vi "FPGA_RTDS_PCC_v02b_clean.vi"() -> ()   [LabVIEW 2015]
uses:
  Analog Measurements Cluster.ctl
  Reactive Power Cluster.ctl
  Real Power Cluster.ctl
  <vilib>/Platform/TimedLoop/XDataNode/timing_clust.ctl
  <vilib>/Platform/TimedLoop/XDataNode/nitl_modes.ctl
  <vilib>/Platform/TimedLoop/XDataNode/wakeup.ctl
  <vilib>/rvi/FXPMathLib/basic elements/FxpIntAccumulator/subVIs/nifxpmath_IntAccumulator_SimConfig.ctl
  <vilib>/rvi/FXPMathLib/FxpSinAndCos/subVIs/nifxpmath_SinAndCos_SimConfig.ctl
  <vilib>/rvi/FXPMathLib/FxpSqrt/subVIs/nifxpmath_Sqrt_SimConfig.ctl
  <vilib>/fxp/LVFixedPointOverflowPolicyTypeDef.ctl
  <vilib>/rvi/Emulation/niFpgaGetClockAttributes.vi
  <vilib>/rvi/Emulation/niFpgaSctlEmulationGetInTimedLoop.vi
  <vilib>/rvi/Emulation/niFpgaEmulationReportErrorSimple.vi
  <vilib>/rvi/eio/common/nirviEmuTemplateMethod_errors.vi
  <vilib>/rvi/Emulation/niFpgaProcessEmulError.vi
  <vilib>/rvi/Emulation/niFpgaCriticalErrorInLSC.vi
  <vilib>/rvi/Analysis/common/codeGenErrors/XNode/niFpgaXNodeCodeGenErrorHandle.vi
  <vilib>/rvi/FXPMathLib/basic elements/FxpIntAccumulator/simVIs/DllFxpIntAccumulator_sub.vi
  <vilib>/rvi/FXPMathLib/FxpSqrt/simVIs/DllSqrtTemp_sub.vi
  <vilib>/rvi/FXPMathLib/FxpSinAndCos/simVIs/DllFxpSinAndCosTemp_sub.vi
  <vilib>/eio/EIONode/EIONode.xnode
  <vilib>/rvi/Analysis/measure/dc-rms/XNode/niFpgaDC-RMS.xnode
  <vilib>/Platform/TimedLoop/XDataNode/XDataNode.xnode
  <vilib>/rvi/FXPMathLib/basic elements/FxpIntAccumulator/XNode/nifxpmath_IntAccumulator.xnode
  <vilib>/rvi/FXPMathLib/FxpMul/XNode/nifxpmath_Multiplier.xnode
  <vilib>/rvi/FXPMathLib/FxpSqrt/XNode/nifxpmath_Sqrt.xnode
  <vilib>/rvi/FXPMathLib/FxpSinAndCos/XNode/nifxpmath_SinAndCos.xnode
  <vilib>/rvi/Analysis/measure/mean-var-std/XNode/niFpgaMean-Var-Std.xnode
  <vilib>/Platform/TimedLoop/XDataNode/XDNodeRunTimeDep.lvlib
  <vilib>/rvi/FXPMathLib/sim/FxpSim.dll
panel:
  in  "close threshold":fxp<+,27,5>=0.09999990463256836 format="%#_24g"
  out "RMS Voltage in Range (resync)":bool
  out "RMS Time":u32
  in  "RMS Loop Time":u32=1500 caption="Count(Ticks)"
  out "Grid I RMS":fxp<+,27,5>
  out "output rms valid":bool
  in  "RMS reset":bool
  in  "Vgrid RMS constant (off grid)":fxp<+,27,5>=0.1399998664855957
  out "Microgrid RMS":fxp<+,27,5>
  out "Grid RMS":fxp<+,27,5>
  out "Mean Computation Valid":bool
  in  "Mean Reset":bool
  out "Phase Diff":fxp<+/-,33,2>
  out "cos(x)":fxp<+/-,16,2>
  out "sin(x)":fxp<+/-,16,2>
  out "Real Power (from mean)":T1
  in  "Computation Loop Time (uSec)":u32=10 caption="Count(uSec)"
  out "Mean Computation Timing Error":bool
  out "Real Power (from angle)":T1
  out "Reactive Power":T2
  in  "Data Acquisition Loop Time (uSec)":u32=10 caption="Count(uSec)"
  out "Data Acquisition Timing Error":bool
  out "Va grid":fxp<+/-,16,5>
  out "Vb grid":fxp<+/-,16,5>
  out "Vc grid":fxp<+/-,16,5>
  out "Ia":fxp<+/-,16,5>
  out "Ib":fxp<+/-,16,5>
  out "Ic":fxp<+/-,16,5>
  out "Phase angle error":fxp<+,32,1>
  out "Freq error":fxp<+,32,8>
  in  "Resync Loop Time":u32=1500 caption="Count(Ticks)"
  out "Resync Time":u32
  in  "Freq constant":fxp<+,32,8>
  out "Switch Closed?":bool
  out "Voltage error\n(on grid)":fxp<+,31,9>
  in  "Enable Resync":bool
  out "Close Switch":bool
  in  "Phase angle constant":fxp<+,32,1>=0.049999999813735485
  out "Open Switch":bool
  in  "MG_SW_constant":fxp<+/-,24,5>=4.0
  in  "Voltage constant (on grid)":fxp<+/-,28,7>=0.26999998092651367
  in  "Vgrid RMS constant (on grid)":fxp<+,27,9>=2.770000457763672
  in  "Enable Switching":bool
  out "Microgrid switch signal":fxp<+/-,24,5>
  in  "Manually Close":bool
  in  "Manually Open":bool
  out "Current\npll phase":fxp<+/-,32,1> format="%.32g"
  out "Current \nfrequency":fxp<+,32,8> format="%.27g"
  in  "PLL Loop Time":u32=1500 caption="Count(Ticks)"
  out "PLL Time MG":u32
  in  "Ki":fxp<+,16,9>=1.0
  in  "Kp":fxp<+,16,6>=0.0146484375
  in  "Ka":fxp<+,16,9>=1.0 format="%#_10g"
  out "Microgrid\npll phase":fxp<+/-,32,1> format="%.32g"
  out "Microgrid \nfrequency":fxp<+,32,8> format="%.27g"
  out "Grid\npll phase":fxp<+/-,32,1> format="%.32g"
  out "Grid \nFrequency":fxp<+,32,8> format="%.27g"
  in  "PLL dt":fxp<+,24,-5>=9.999983012676239e-05 format="%#_28g"
  in  "Reset PLL":bool
  in  "LPF Alpha":sgl[](array[numeric])=[0.19, 0.19, 0.19, 0.1, 0.1, 0.1, 0.1, 0.1, 0.1]
  in  "LPF enable":bool=TRUE
  out "Grid Iabc":T3
  out "Grid Vabc":T4
  out "Microgrid Vabc":T4
  in  "Count(Ticks)":u32=1500
  out "Loop rate":u32
  out "RMS Computation Valid":bool
  out "RMS Computation Timing Error":bool
  out "Analog rms output":T5
  # "Logic RMS Computation"
  # "Power Computation"
  # "Data Acquisition"
  # "RMS Computation"
  # "PLL Calculations"
  # "Low Pass Filter"
  # "RMS Computation"
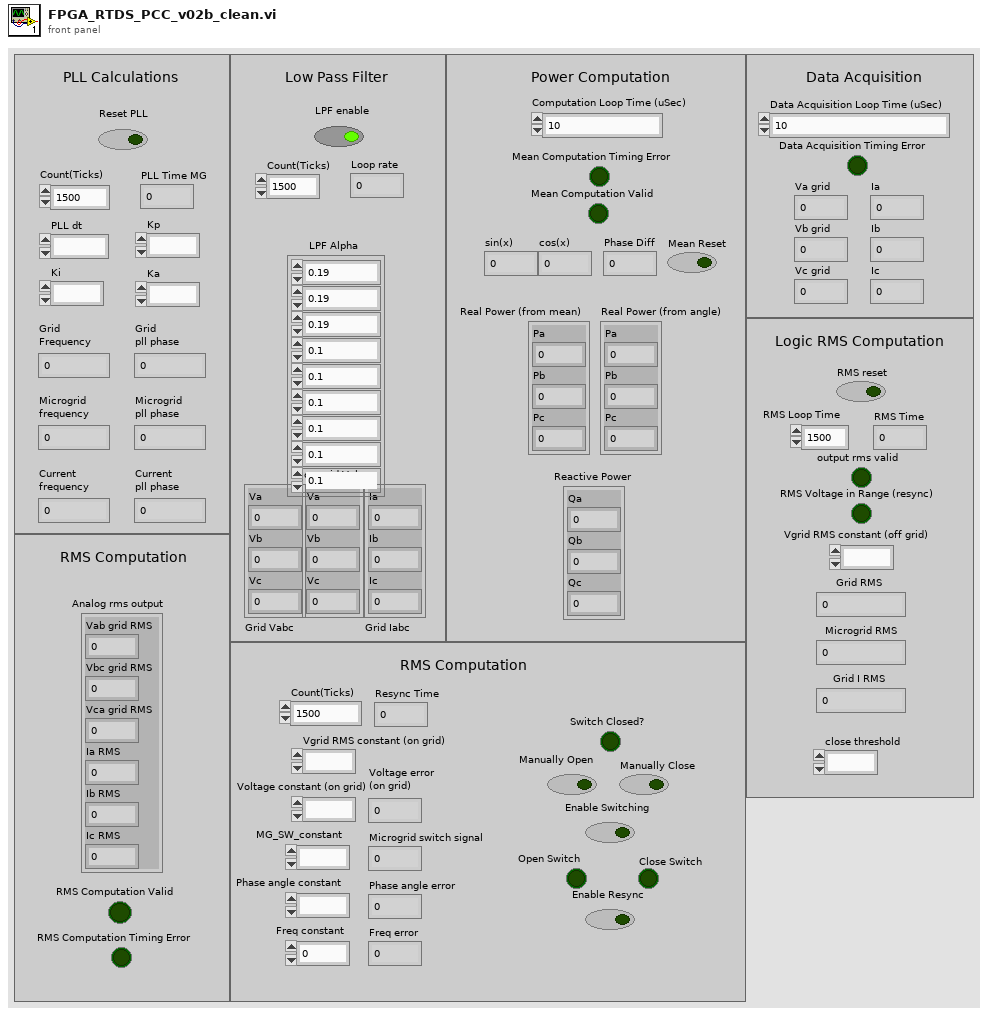
[diagram p1: front panel]
types:
  T1 = typedef "Real Power Cluster.ctl" = cluster{"Pa":fxp<+/-,32,10>, "Pb":fxp<+/-,32,10>, "Pc":fxp<+/-,32,10>}
  T2 = typedef "Reactive Power Cluster.ctl" = cluster{"Qa":fxp<+/-,46,10>, "Qb":fxp<+/-,46,10>, "Qc":fxp<+/-,46,10>}
  T3 = cluster{"Ia":fxp<+/-,24,5>, "Ib":fxp<+/-,24,5>, "Ic":fxp<+/-,24,5>}
  T4 = cluster{"Va":fxp<+/-,18,4>, "Vb":fxp<+/-,18,4>, "Vc":fxp<+/-,18,4>}
  T5 = typedef "Analog Measurements Cluster.ctl" = cluster{"Vab grid RMS":fxp<+,16,5>, "Vbc grid RMS":fxp<+,16,5>, "Vca grid RMS":fxp<+,16,5>, "Ia RMS":fxp<+,16,5>, "Ib RMS":fxp<+,16,5>, "Ic RMS":fxp<+,16,5>}
  T6 = typedef "XDNodeRunTimeDep.lvlib/timing_clust.ctl" = cluster{"Expected End [f-1]":u64, "Actual End [f-1]":u64, "Finished Late? [f-1]":bool, "Expected End [i-1]":u64, "Actual End [i-1]":u64, "Finished Late? [i-1]":bool, "Expected Start [i]":u64, "Actual Start [i]":u64, "Expected Start [f]":u64, "Actual Start [f]":u64, "Source Name":string, "Structure Name":string, "Period":i64, "Deadline":i64, "Offset":i64, "Start":i64, "Priority":i32, "Timeout":i32, "Mode":T7, "Wakeup Reason":T8, "Error":errorcluster, "Source Type":string, "Secondary Source Type":string, "Global End Time":u64, "Global Start Time":u64, "Frame Duration":u64, "Iteration Duration":u64, "Assigned CPU":i32, "I/O Scan Engine Mode":u32}
  T7 = typedef "XDNodeRunTimeDep.lvlib/nitl_modes.ctl" = enum32{"No Change", "Process missed periods, maintain original phase", "Discard missed periods, maintain original phase", "Process missed periods, ignore original phase", "Discard missed periods, ignore original phase"}
  T8 = typedef "XDNodeRunTimeDep.lvlib/wakeup.ctl" = enum32{"Normal", "Aborted", "Asynchronous wakeup", "Timing source error", "Timed loop error", "Timeout"}
  T9 = cluster{"filtered x":sgl, "filtered x":sgl, "filtered x":sgl}
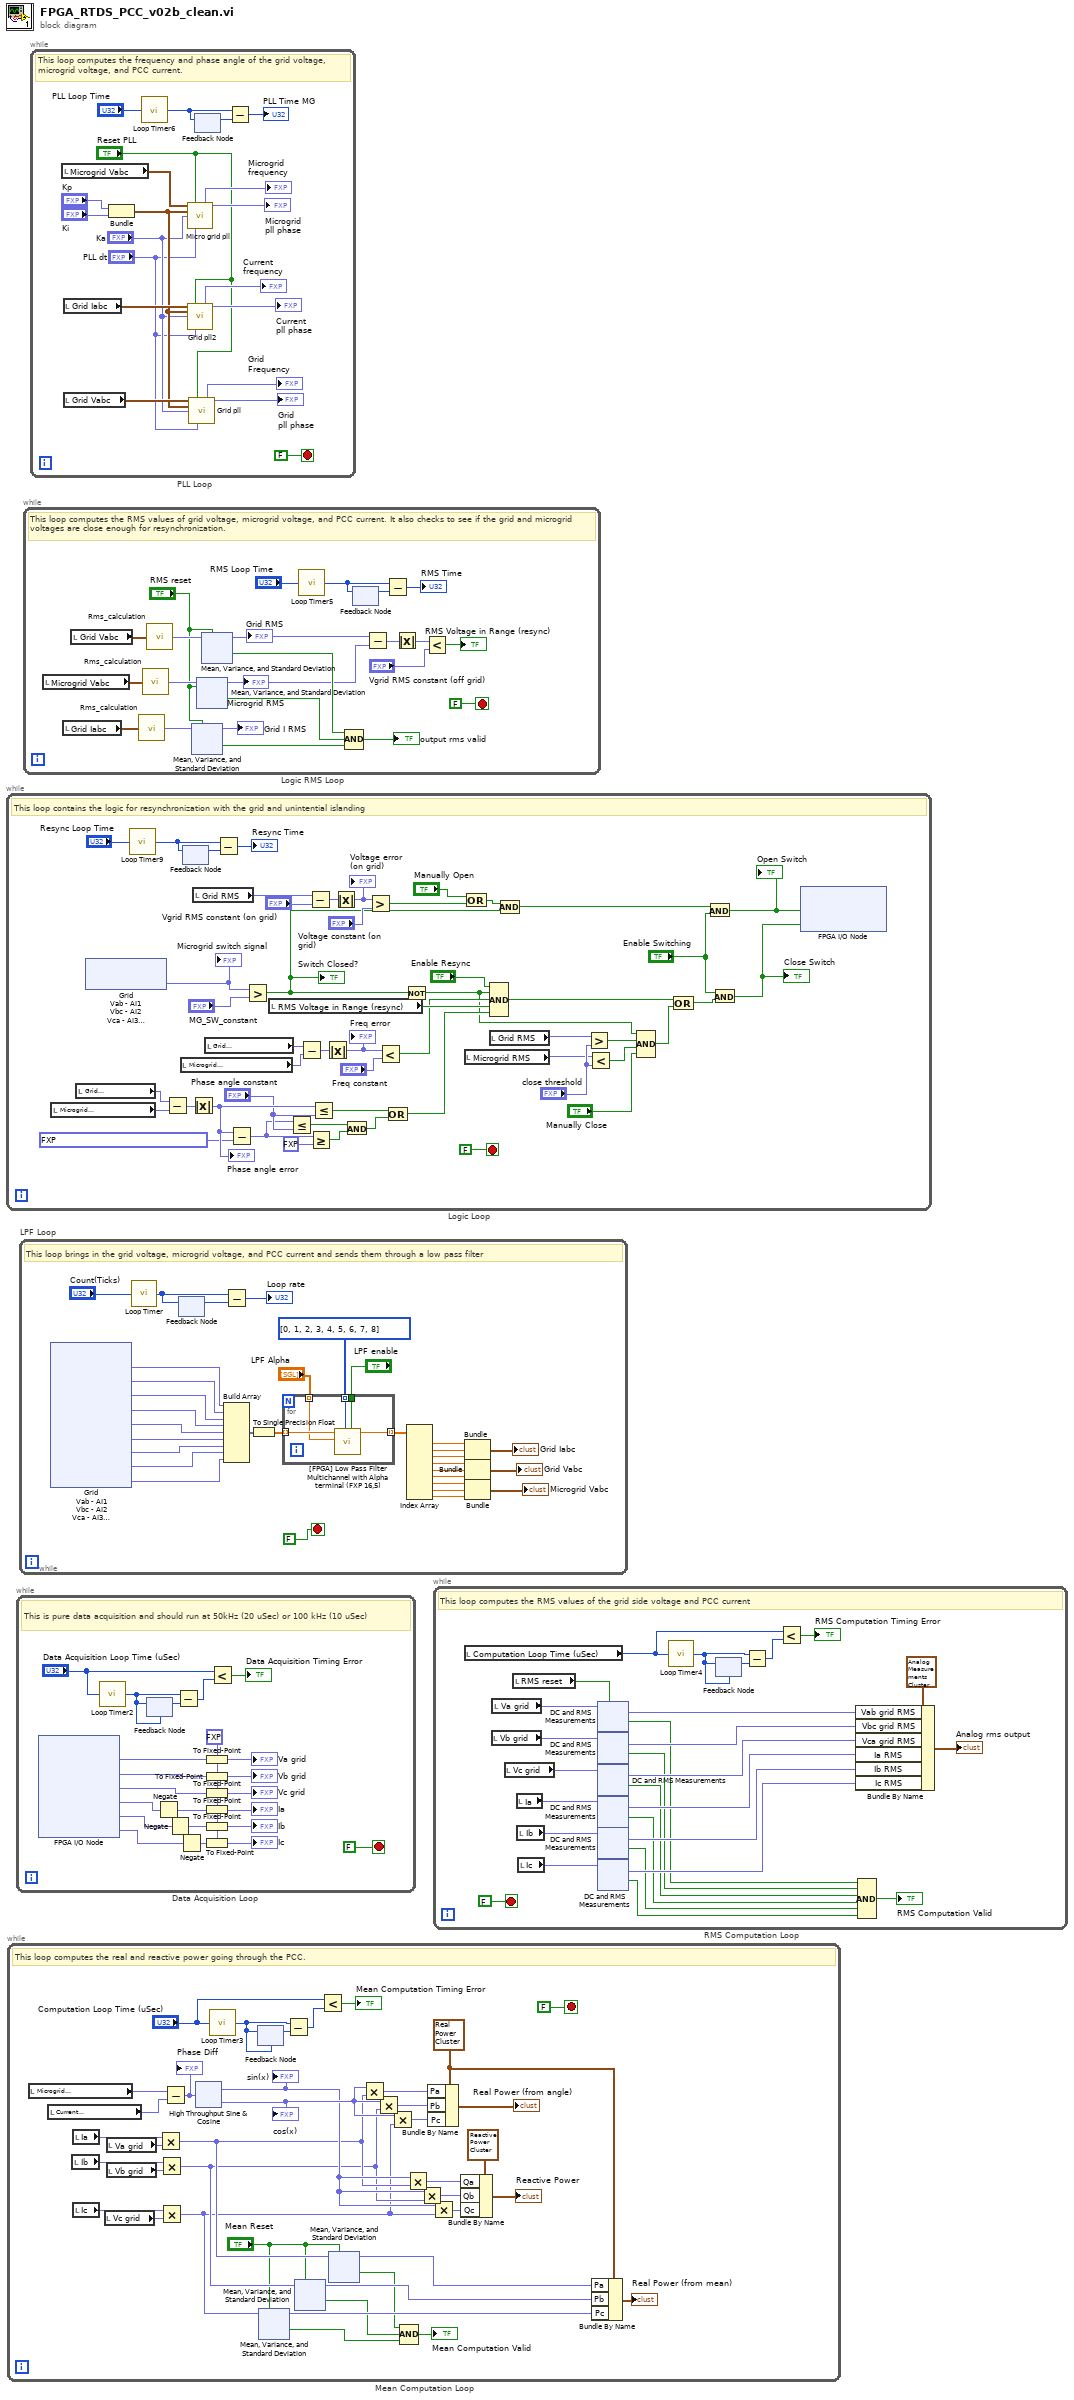
[diagram p0: block diagram]
diagram:
  n1 = while "Logic Loop" {
    stop <- FALSE stop-if-true
    # "This loop contains the logic for resynchronization with the grid and unintential islanding"
    n2 = local read "Microgrid\npll phase"() -> (w35:fxp<+/-,32,1>)
    n3 = local read "Grid\npll phase"() -> (w34:fxp<+/-,32,1>)
    n4 = xnode ("Grid \nVab - AI1\nVbc - AI2\nVca - AI3\nIa - AI7\nIb - AI8\nIc - AI9")() -> ("Mod1/AI0"=w27:fxp<+/-,24,5>)  [unwired: 1 in, 1 out]
    "Microgrid switch signal" <- w27
    n5 = call "Loop Timer9"("Count(Ticks)"="Resync Loop Time") -> ("Tick Count(Ticks)"=w21:u32)
    n6 = Subtract(x=w34, y=w35) -> (x-y=w45:fxp<+/-,33,2>)
    n7 = local read "Microgrid \nfrequency"() -> (w46:fxp<+,32,8>)
    n8 = feedback #1() -> (w20:u32)  [unwired: 1 in]
    n9 = feedback-in #1(w21) -> ()
    n10 = Absolute Value(x=w45) -> (abs(x)=w44:fxp<+,32,1>)
    "Phase angle error" <- w44
    n11 = local read "Grid RMS"() -> (w26:fxp<+,27,5>)
    n12 = local read "Grid \nFrequency"() -> (w47:fxp<+,32,8>)
    n13 = Subtract(x=w21, y=w20) -> (x-y=→"Resync Time":u32)
    n14 = Subtract(x=w44, y=fxp<+,32,1> 1.9999999995343387) -> (x-y=w41:fxp<+/-,33,2>)
    n15 = Greater?(x=w27, y="MG_SW_constant") -> (0:w28:bool)
    "Switch Closed?" <- w28
    n16 = local read "RMS Voltage in Range (resync)"() -> (w24:bool)
    n17 = Less Or Equal?(x=w41, y="Phase angle constant") -> (x <= y?=w39:bool)
    n18 = Subtract(x=w47, y=w46) -> (x-y=w50:fxp<+/-,33,9>)
    n19 = Subtract(x=w26, y="Vgrid RMS constant (on grid)") -> (x-y=w32:fxp<+/-,32,10>)
    n20 = Greater Or Equal?(x=w41, y=fxp<+/-,33,2> 0.0) -> (x >= y?=w38:bool)
    n21 = Less Or Equal?(x=w44, y="Phase angle constant") -> (x <= y?=w37:bool)
    n22 = Absolute Value(x=w50) -> (abs(x)=w49:fxp<+,32,8>)
    "Freq error" <- w49
    n23 = Absolute Value(x=w32) -> (abs(x)=w30:fxp<+,31,9>)
    "Voltage error\n(on grid)" <- w30
    n24 = Compound Arithmetic op=AND(w39, w38) -> (w36:bool)
    n25 = Greater?(x=w30, y="Voltage constant (on grid)") -> (0:w18:bool)
    n26 = Less?(x=w49, y="Freq constant") -> (x < y?=w23:bool)
    n27 = Compound Arithmetic op=OR(w37, w36) -> (w25:bool)
    n28 = Not(x=w28) -> (.not. x?=w1:bool)
    n29 = local read "Microgrid RMS"() -> (w6:fxp<+,27,5>)
    n30 = Compound Arithmetic op=OR("Manually Open", w18) -> (w17:bool)
    n31 = Compound Arithmetic op=AND("Enable Resync", w1, w23, w24, w25) -> (w10:bool)
    n32 = local read "Grid RMS"() -> (w8:fxp<+,27,5>)
    n33 = Compound Arithmetic op=AND(w17, w28) -> (w15:bool)
    n34 = Greater?(x=w8, y="close threshold") -> (0:w5:bool)
    n35 = Less?(x=w6, y="close threshold") -> (x < y?=w4:bool)
    n36 = Compound Arithmetic op=AND(w1, w5, w4, "Manually Close") -> (w2:bool)
    n37 = Compound Arithmetic op=OR(w10, w2) -> (w9:bool)
    n38 = And(x=w15, y="Enable Switching") -> (x .and. y?=w13:bool)
    "Open Switch" <- w13
    n39 = And(x="Enable Switching", y=w9) -> (x .and. y?=w12:bool)
    "Close Switch" <- w12
    n40 = xnode "FPGA I/O Node"("Mod3/DO0"=w13, "Mod3/DO1"=w12) -> ()  [unwired: 2 in, 2 out]
  }
  n41 = while "Mean Computation Loop" {
    stop <- FALSE stop-if-true
    w61 = T1 {"Pa"=0.0, "Pb"=0.0, "Pc"=0.0} ("output cluster")
    # "This loop computes the real and reactive power going through the PCC."
    n42 = local read "Microgrid\npll phase"() -> (w77:fxp<+/-,32,1>)
    n43 = local read "Current\npll phase"() -> (w76:fxp<+/-,32,1>)
    n44 = local read "Ib"() -> (w88:fxp<+/-,16,5>)
    n45 = local read "Ia"() -> (w89:fxp<+/-,16,5>)
    n46 = local read "Ic"() -> (w85:fxp<+/-,16,5>)
    n47 = local read "Vc grid"() -> (w86:fxp<+/-,16,5>)
    n48 = local read "Va grid"() -> (w90:fxp<+/-,16,5>)
    n49 = local read "Vb grid"() -> (w87:fxp<+/-,16,5>)
    n50 = Multiply(x=w89, y=w90) -> (x*y=w64:fxp<+/-,32,10>)
    n51 = Multiply(x=w88, y=w87) -> (x*y=w63:fxp<+/-,32,10>)
    n52 = Multiply(x=w85, y=w86) -> (x*y=w62:fxp<+/-,32,10>)
    n53 = Subtract(x=w77, y=w76) -> (x-y=w75:fxp<+/-,33,2>)
    "Phase Diff" <- w75
    n54 = xnode "High Throughput Sine & Cosine"("x (pi)"=w75) -> ("sin(x)"=w67:fxp<+/-,16,2>, "cos(x)"=w71:fxp<+/-,16,2>)
    "sin(x)" <- w67
    "cos(x)" <- w71
    n55 = call "Loop Timer3"("Count(uSec)"="Computation Loop Time (uSec)") -> ("Tick Count(uSec)"=w80:u32)
    n56 = feedback #2(w80) -> (w79:u32)
    n57 = feedback-in #2(w80) -> ()
    n58 = xnode "Mean, Variance, and Standard Deviation"("input data"=w62, "reset"="Mean Reset") -> ("mean"=w58:fxp<+/-,32,10>, "output valid"=w56:bool)
    n59 = Subtract(x=w80, y=w79) -> (x-y=w82:u32)
    n60 = xnode "Mean, Variance, and Standard Deviation"("input data"=w63, "reset"="Mean Reset") -> ("mean"=w59:fxp<+/-,32,10>, "output valid"=w54:bool)
    n61 = Less?(x="Computation Loop Time (uSec)", y=w82) -> (x < y?=→"Mean Computation Timing Error":bool)
    n62 = xnode "Mean, Variance, and Standard Deviation"("input data"=w64, "reset"="Mean Reset") -> ("mean"=w60:fxp<+/-,32,10>, "output valid"=w53:bool)
    n63 = Multiply(x=w71, y=w64) -> (x*y=w72:fxp<+/-,46,10>)
    n64 = Multiply(x=w71, y=w63) -> (x*y=w73:fxp<+/-,46,10>)
    n65 = Multiply(x=w71, y=w62) -> (x*y=w74:fxp<+/-,46,10>)
    n66 = Compound Arithmetic op=AND(w53, w54, w56) -> (→"Mean Computation Valid":bool)
    n67 = Multiply(x=w67, y=w64) -> (x*y=w68:fxp<+/-,46,10>)
    n68 = Multiply(x=w67, y=w63) -> (x*y=w70:fxp<+/-,46,10>)
    n69 = Bundle By Name(cluster=w61, "Pa"=w72, "Pb"=w73, "Pc"=w74) -> (→"Real Power (from angle)":T1)
    n70 = Multiply(x=w67, y=w62) -> (x*y=w69:fxp<+/-,46,10>)
    n71 = Bundle By Name(cluster=T2 {"Qa"=0.0, "Qb"=0.0, "Qc"=0.0} ("input cluster"), "Qa"=w68, "Qb"=w70, "Qc"=w69) -> (→"Reactive Power":T2)
    n72 = Bundle By Name(cluster=w61, "Pa"=w60, "Pb"=w59, "Pc"=w58) -> (→"Real Power (from mean)":T1)
  }
  n73 = while "Data Acquisition Loop" {
    stop <- FALSE stop-if-true
    w352 = fxp<+/-,16,5> 0.0 ("x*y")
    # "This is pure data acquisition and should run at 50kHz (20 uSec) or 100 kHz (10 uSec)"
    n74 = xnode "FPGA I/O Node"() -> ("Mod1/AI1"=w364:fxp<+/-,24,5>, "Mod1/AI2"=w363:fxp<+/-,24,5>, "Mod1/AI3"=w362:fxp<+/-,24,5>, "Mod1/AI7"=w361:fxp<+/-,24,5>, "Mod1/AI8"=w360:fxp<+/-,24,5>, "Mod1/AI9"=w359:fxp<+/-,24,5>)  [unwired: 6 in, 6 out]
    n75 = call "Loop Timer2"("Count(uSec)"="Data Acquisition Loop Time (uSec)") -> ("Tick Count(uSec)"=w369:u32)
    n76 = feedback #3(w369) -> (w370:u32)
    n77 = feedback-in #3(w369) -> ()
    n78 = Negate(x=w361) -> (-x=w351:fxp<+/-,25,6>)
    n79 = Negate(x=w360) -> (-x=w350:fxp<+/-,25,6>)
    n80 = Subtract(x=w369, y=w370) -> (x-y=w367:u32)
    n81 = Negate(x=w359) -> (-x=w349:fxp<+/-,25,6>)
    n82 = To Fixed-Point(fixed-point type=w352, number=w364) -> (fixed-point=→"Va grid":fxp<+/-,16,5>)
    n83 = To Fixed-Point(fixed-point type=w352, number=w363) -> (fixed-point=→"Vb grid":fxp<+/-,16,5>)
    n84 = To Fixed-Point(fixed-point type=w352, number=w362) -> (fixed-point=→"Vc grid":fxp<+/-,16,5>)
    n85 = To Fixed-Point(fixed-point type=w352, number=w351) -> (fixed-point=→"Ia":fxp<+/-,16,5>)
    n86 = To Fixed-Point(fixed-point type=w352, number=w350) -> (fixed-point=→"Ib":fxp<+/-,16,5>)
    n87 = To Fixed-Point(fixed-point type=w352, number=w349) -> (fixed-point=→"Ic":fxp<+/-,16,5>)
    n88 = Less?(x="Data Acquisition Loop Time (uSec)", y=w367) -> (x < y?=→"Data Acquisition Timing Error":bool)
  }
  n89 = while "LPF Loop" {
    stop <- FALSE ("stop") stop-if-true
    # "This loop brings in the grid voltage, microgrid voltage, and PCC current and sends them through a low pass filter"
    n90 = xnode ("Grid \nVab - AI1\nVbc - AI2\nVca - AI3\nIa - AI7\nIb - AI8\nIc - AI9")() -> ("Mod1/AI7"=w373:fxp<+/-,24,5>, "Mod1/AI8"=w372:fxp<+/-,24,5>, "Mod1/AI9"=w371:fxp<+/-,24,5>, "Mod1/AI1"=w390:fxp<+/-,24,5>, "Mod1/AI2"=w389:fxp<+/-,24,5>, "Mod1/AI3"=w388:fxp<+/-,24,5>, "Mod1/AI4"=w387:fxp<+/-,24,5>, "Mod1/AI5"=w386:fxp<+/-,24,5>, "Mod1/AI6"=w385:fxp<+/-,24,5>)  [unwired: 9 in, 9 out]
    n91 = call "Loop Timer"("Count(Ticks)"="Count(Ticks)") -> ("Tick Count(Ticks)"=w401:u32)
    n92 = feedback #4() -> (w400:u32)  [unwired: 1 in]
    n93 = feedback-in #4(w401) -> ()
    n94 = Subtract(x=w401, y=w400) -> (x-y=→"Loop rate":u32)
    n95 = Build Array(w373, w372, w371, w390, w389, w388, w387, w386, w385) -> (w391:fxp<+/-,24,5>[])
    n96 = To Single Precision Float(number=w391) -> (single precision float=w384:sgl[])
    n97 = for {
      tunnel: w384 -> [w407] mode=indexing
      tunnel: "LPF Alpha" -> [w406] mode=indexing
      tunnel: "LPF enable" -> [w405]
      tunnel: [w404] -> w383 mode=indexing
      tunnel: u32[] [0, 1, 2, 3, 4, 5, 6, 7, 8] -> [w403] mode=indexing
      n98 = call "[FPGA] Low Pass Filter Multichannel with Alpha terminal (FXP 16,5).vi"("enable"=w405, "Channel #"=w403, "LPF alpha"=w406, "x"=w407) -> ("filtered x"=w404:sgl)  [unwired: 7 in]
    }
    n99 = Index Array(array=w383) -> (element #1=w382:sgl, element #2=w381:sgl, element #3=w380:sgl, element #4=w379:sgl, element #5=w378:sgl, element #6=w377:sgl, element #7=w376:sgl, element #8=w375:sgl, element #9=w374:sgl)  [unwired: 9 in]
    n100 = Bundle ("Grid \ncurrent\n bundle")("filtered x"=w382, "filtered x"=w381, "filtered x"=w380) -> (→"Grid Iabc":T9)  [unwired: 1 in]
    n101 = Bundle ("Grid \nvoltage\n bundle")("filtered x"=w379, "filtered x"=w378, "filtered x"=w377) -> (→"Grid Vabc":T9)  [unwired: 1 in]
    n102 = Bundle ("Microgrid\nvoltage bundle")("filtered x"=w376, "filtered x"=w375, "filtered x"=w374) -> (→"Microgrid Vabc":T9)  [unwired: 1 in]
  }
  n103 = while "Logic RMS Loop" {
    stop <- FALSE stop-if-true
    # "This loop computes the RMS values of grid voltage, microgrid voltage, and PCC current. It also checks to see if the grid and microgrid voltages are close enough for resynchronization."
    n104 = local read "Microgrid Vabc"() -> (w420:T4)
    n105 = local read "Grid Iabc"() -> (w427:T3)
    n106 = local read "Grid Vabc"() -> (w425:T4)
    n107 = call "Rms_calculation.vi"("Vabc"=w427) -> ("Three phase RMS"=w428:fxp<+,27,5>)
    n108 = call "Rms_calculation.vi"("Vabc"=w420) -> ("Three phase RMS"=w424:fxp<+,27,5>)
    n109 = call "Rms_calculation.vi"("Vabc"=w425) -> ("Three phase RMS"=w426:fxp<+,27,5>)
    n110 = xnode "Mean, Variance, and Standard Deviation"("input data"=w428, "reset"="RMS reset") -> ("mean"=→"Grid I RMS":fxp<+,27,5>, "output valid"=w421:bool)
    n111 = xnode "Mean, Variance, and Standard Deviation"("input data"=w424, "reset"="RMS reset") -> ("mean"=w409:fxp<+,27,5>, "output valid"=w412:bool)
    "Microgrid RMS" <- w409
    n112 = xnode "Mean, Variance, and Standard Deviation"("input data"=w426, "reset"="RMS reset") -> ("mean"=w410:fxp<+,27,5>, "output valid"=w411:bool)
    "Grid RMS" <- w410
    n113 = call "Loop Timer5"("Count(Ticks)"="RMS Loop Time") -> ("Tick Count(Ticks)"=w417:u32)
    n114 = Compound Arithmetic op=AND(w411, w412, w421) -> (→"output rms valid":bool)
    n115 = feedback #5() -> (w418:u32)  [unwired: 1 in]
    n116 = feedback-in #5(w417) -> ()
    n117 = Subtract(x=w410, y=w409) -> (x-y=w415:fxp<+/-,28,6>)
    n118 = Subtract(x=w417, y=w418) -> (x-y=→"RMS Time":u32)
    n119 = Absolute Value(x=w415) -> (abs(x)=w414:fxp<+,27,5>)
    n120 = Less?(x=w414, y="Vgrid RMS constant (off grid)") -> (x < y?=→"RMS Voltage in Range (resync)":bool)
  }
  n121 = while "PLL Loop" {
    stop <- FALSE stop-if-true
    # "This loop computes the frequency and phase angle of the grid voltage, microgrid voltage, and PCC current."
    n122 = local read "Microgrid Vabc"() -> (w671:T4)
    n123 = local read "Grid Iabc"() -> (w666:T3)
    n124 = local read "Grid Vabc"() -> (w663:T4)
    n125 = Bundle("Kp"="Kp", "Ki"="Ki") -> (w662:cluster{"Kp":fxp<+,16,6>, "Ki":fxp<+,16,9>})  [unwired: 1 in]
    n126 = call "Loop Timer6"("Count(Ticks)"="PLL Loop Time") -> ("Tick Count(Ticks)"=w675:u32)
    n127 = call "Micro grid pll"("input (phase value)"=w671, "reset"="Reset PLL", "PI gains"=w662, "anti-windup gain (Ka)"="Ka", "dt"="PLL dt") -> ("frequency"=→"Microgrid \nfrequency":fxp<+,32,8>, "phase (pi)"=→"Microgrid\npll phase":fxp<+/-,32,1>)  [unwired: 7 in, 2 out]
    n128 = call "Grid pll2"("input (phase value)"=w666, "reset"="Reset PLL", "PI gains"=w662, "anti-windup gain (Ka)"="Ka", "dt"="PLL dt") -> ("frequency"=→"Current \nfrequency":fxp<+,32,8>, "phase (pi)"=→"Current\npll phase":fxp<+/-,32,1>)  [unwired: 7 in, 2 out]
    n129 = call "Grid pll"("input (phase value)"=w663, "reset"="Reset PLL", "PI gains"=w662, "anti-windup gain (Ka)"="Ka", "dt"="PLL dt") -> ("frequency"=→"Grid \nFrequency":fxp<+,32,8>, "phase (pi)"=→"Grid\npll phase":fxp<+/-,32,1>)  [unwired: 7 in, 2 out]
    n130 = feedback #6() -> (w676:u32)  [unwired: 1 in]
    n131 = feedback-in #6(w675) -> ()
    n132 = Subtract(x=w675, y=w676) -> (x-y=→"PLL Time MG":u32)
  }
  n133 = while "RMS Computation Loop" {
    stop <- FALSE stop-if-true
    # "This loop computes the RMS values of the grid side voltage and PCC current"
    n134 = local read "Computation Loop Time (uSec)"() -> (w697:u32)
    n135 = local read "Vb grid"() -> (w705:fxp<+/-,16,5>)
    n136 = local read "Va grid"() -> (w706:fxp<+/-,16,5>)
    n137 = local read "Vc grid"() -> (w704:fxp<+/-,16,5>)
    n138 = local read "RMS reset"() -> (w679:bool)
    n139 = local read "Ia"() -> (w703:fxp<+/-,16,5>)
    n140 = local read "Ib"() -> (w702:fxp<+/-,16,5>)
    n141 = local read "Ic"() -> (w701:fxp<+/-,16,5>)
    n142 = xnode "DC and RMS Measurements"("input data"=w706, "reset"=w679) -> ("RMS"=w692:fxp<+,16,5>, "output valid"=w681:bool)
    n143 = xnode "DC and RMS Measurements"("input data"=w705, "reset"=w679) -> ("RMS"=w691:fxp<+,16,5>, "output valid"=w682:bool)
    n144 = xnode "DC and RMS Measurements"("input data"=w704, "reset"=w679) -> ("RMS"=w690:fxp<+,16,5>, "output valid"=w683:bool)
    n145 = xnode "DC and RMS Measurements"("input data"=w703, "reset"=w679) -> ("RMS"=w689:fxp<+,16,5>, "output valid"=w684:bool)
    n146 = xnode "DC and RMS Measurements"("input data"=w702, "reset"=w679) -> ("RMS"=w688:fxp<+,16,5>, "output valid"=w685:bool)
    n147 = xnode "DC and RMS Measurements"("input data"=w701, "reset"=w679) -> ("RMS"=w687:fxp<+,16,5>, "output valid"=w686:bool)
    n148 = call "Loop Timer4"("Count(uSec)"=w697) -> ("Tick Count(uSec)"=w699:u32)
    n149 = feedback #7(w699) -> (w700:u32)
    n150 = feedback-in #7(w699) -> ()
    n151 = Subtract(x=w699, y=w700) -> (x-y=w698:u32)
    n152 = Less?(x=w697, y=w698) -> (x < y?=→"RMS Computation Timing Error":bool)
    n153 = Bundle By Name(cluster=T5 {"Vab grid RMS"=0.0, "Vbc grid RMS"=0.0, "Vca grid RMS"=0.0, "Ia RMS"=0.0, "Ib RMS"=0.0, "Ic RMS"=0.0} ("output cluster"), "Vab grid RMS"=w692, "Vbc grid RMS"=w691, "Vca grid RMS"=w690, "Ia RMS"=w689, "Ib RMS"=w688, "Ic RMS"=w687) -> (→"Analog rms output":T5)
    n154 = Compound Arithmetic op=AND(w681, w682, w683, w684, w685, w686) -> (→"RMS Computation Valid":bool)
  }
